vi "PCO_GetCameraDescription.vi"(8 "error in (no error)":errorcluster, 11 "Handle":u32=176713696) -> (0 "error out":errorcluster, 1 "PCO_Description_part2":T1={"wIRDESC"=1, "ZZwAlignDummy2"=0, "dwMinDelay[ns]"=0, "dwMaxDelay[ms]"=0, "dwMinDelayStep[ns]"=100, "dwMinExposure[ns]"=1000, "dwMaxExposure[ms]"=3600000, "dwMinExposureStep[ns]"=1000, "dwMinDelay[ns]"=0, "dwMaxDelay[ms]"=0, "dwMinExposureIR[ns]"=1000, "dwMaxExposureIR[ms]"=3600000, "wTimeTableDESC"=0, "wDoubleImageDESC"=1, "sMinCoolSetDESC"=0, "sMaxCoolSetDESC"=1, "sDefaultCoolSetDESC"=0, "wPowerDownModeDESC"=0, "wOffsetRegulationDESC"=1, "wColorPatternDESC"=0, "wPatternTypeDESC"=0, "wDummy1"=0, "wDummy2"=0, "wDummy3"=0, "dwGeneralCapsDESC1"=64, "dwGeneralCapsDESC2"=0}, 2 "PCO_Description_part1":T2={"wSensorTypeDESC"=16, "wSensorSubTypeDESC"=0, "wMaxHorzResStdDESC"=1392, "wMaxVertResStdDESC"=1040, "wMaxHorzResExtDESC"=800, "wMaxVertResExtDESC"=600, "wDynRes[bits]"=14, "wMaxBinHorzDESC"=4, "wBinHorzSteppingDESC"=0, "wMaxBinVertDESC"=4, "wBinVertSteppingDESC"=0, "wRoiHorStepsDESC"=0, "wRoiVertStepsDESC"=0, "wNumADCsDESC"=1} {"wSensorTypeDESC" items=["Sony ICX285AL"=16, "Sony ICX285AK"=17, "Sony ICX263AL"=32, "Sony ICX263AK"=33, "Sony ICX274AL"=48, "Sony ICX274AK"=49, "Sony ICX407AL"=64, "Sony ICX407AK"=65, "Sony ICX414AL"=80, "KAI-2000M"=272, "KAI-2001M"=288, "KAI-4010M"=304, "KAI-4011M"=306, "Micron MV13 bw"=4112, "Micron MV13 col"=4113, "Fairchild CIS2051 V1 FI"=8192, "Fairchild CIS2051 V1 BI"=8208, "Cypress RR V1 bw"=12288, "Cypress RR V1 col"=12289]}, 3 "Handle Out":u32=176713696, 4 "wConvFact[ce]":u16[](array[numeric])=[100, 150, 0, 0], 5 "return type":u32 format="%x", 6 "dwPixelRate[Hz]":u32[](array[numeric])=[12000000, 25000000, 0, 0])   [LabVIEW 2011]
uses:
  SC2_Cam64.dll
panel:
  out "PCO_Description":u16[](array[numeric])=[436, 16, 0, 1392, 1040, 800, 600, 14, 4, 0, 4, 0, 0, 0, 1, 0, 6912, 183, 30784, 381, 0, 0, 0, 0, 0, 0, 0, 0, 0, 0, 0, 0, 0, 0, 0, 0, 0, 0, 0, 0, 0, 0, 0, 0, 0, 0, 0, 0, 0, 0, 0, 0, 0, 0, 0, 0, 0, 0, 0, 0, 0, 0, 0, 0, 100, 150, 0, 0, 0, 0, 0, 0, 0, 0, 0, 0, 0, 0, 0, 0, 0, 0, 0, 0, 0, 0, 0, 0, 1, 0, 0, 0, 0, 0, 100, 0, 1000, 0, 61056, 54, 1000, 0, 0, 0, 0, 0, 1000, 0, 61056, 54, 0, 1, 0, 1, 0, 0, 1, 0, 0, 0, 0, 0, 64, 0, 0, 0, 0, 0, 0, 0, 0, 0, 0, 0, 0, 0, 0, 0, 0, 0, 0, 0, 0, 0, 0, 0, 0, 0, 0, 0, 0, 0, 0, 0, 0, 0, 0, 0, 0, 0, 0, 0, 0, 0, 0, 0, 0, 0, 0, 0, 0, 0, 0, 0, 0, 0, 0, 0, 0, 0, 0, 0, 0, 0, 0, 0, 0, 0, 0, 0, 0, 0, 0, 0, 0, 0, 0, 0, 0, 0, 0, 0, 0, 0, 0, 0, 0, 0, 0, 0, 0, 0, 0, 0, 0, 0, 0, 0, 0, 0, 0, 0, 0, 0, 0, 0, 0, 0, 0, 0, 0, 0, 0, 0, 0, 0, 0, 0, 0, 0, 0, 0, 0, 0, 0, 0, 0, 0, 0, 0, 0, 0, 0, 0, 0, 0, 0, 0, 0, 0, 0, 0, 0, 0, 0, 0, 0, 0, 0, 0, 0, 0, 0, 0, 0, 0, 0, 0, 0, 0, 0, 0, 0, 0, 0, 0, 0, 0, 0, 0, 0, 0, 0, 0, 0, 0, 0, 0, 0, 0, 0, 0, 0, 0, 0, 0, 0, 0, 0, 0, 0, 0, 0, 0, 0, 0, 0, 0, 0, 0, 0, 0, 0, 0, 0, 0, 0, 0, 0, 0, 0, 0, 0, 0, 0, 0, 0, 0, 0, 0, 0, 0, 0, 0, 0, 0, 0, 0, 0, 0, 0, 0, 0, 0, 0, 0, 0, 0, 0, 0, 0, 0, 0, 0, 0, 0, 0, 0, 0, 0, 0, 0, 0, 0, 0, 0, 0, 0, 0, 0, 0, 0, 0, 0, 0, 0, 0, 0, 0, 0, 0, 0, 0, 0, 0, 0, 0, 0, 0, 0, 0, 0, 0, 0, 0, 0, 0, 0, 0, 0, 0, 0, 0, 0, 0, 0, 0, 0, 0, 0, 0, 0, 0, 0, 0, 0, 0, 0, 0, 0, 0, 0, 0, 0, 0, 0, 0, 0, 0, 0, 0, 0, 0, 0, 0, 0, 0, 0, 0, 0, 0, 0, 0, 0, 0, 0, 0, 0, 0, 0, 0, 0, 0, 0, 0, 0, 0, 0, 0, 0, 0, 0, 0, 0, 0, 0, 0, 0, 0, 0, 0, 0, 0, 0, 0, 0, 0, 0, 0, 0, 0, 0, 0, 0, 0, 0, 0, 0, 0, 0, 0, 0, 0, 0, 0, 0, 0, 0, 0, 0, 0, 0, 0, 0, 0, 0, 0, 0, 0, 0, 0, 0, 0, 0, 0, 0, 0, 0, 0, 0, 0, 0, 0, 0, 0, 0, 0, 0, 0, 0, 0, 0, 0, 0, 0, 0, 0, 0, 0, 0, 0, 0, 0, 0, 0, 0, 0, 0, 0, 0, 0, 0, 0, 0, 0, 0, 0, 0, 0, 0, 0, 0, 0, 0, 0, 0, 0, 0, 0, 0, 0, 0, 0, 0, 0, 0, 0, 0, 0, 0, 0, 0, 0, 0, 0, 0, 0, 0, 0, 0, 0, 0, 0, 0, 0, 0, 0, 0, 0, 0, 0, 0, 0, 0, 0, 0, 0, 0, 0, 0, 0, 0, 0, 0, 0, 0, 0, 0, 0, 0, 0, 0, 0, 0, 0, 0, 0, 0, 0, 0, 0, 0, 0, 0, 0, 0, 0, 0, 0, 0, 0, 0, 0, 0, 0, 0, 0, 0, 0, 0, 0, 0, 0, 0, 0, 0, 0, 0, 0, 0, 0, 0, 0, 0, 0, 0, 0, 0, 0, 0, 0, 0, 0, 0, 0, 0, 0, 0, 0, 0, 0, 0, 0, 0, 0, 0, 0, 0, 0, 0, 0, 0, 0, 0, 0, 0, 0, 0, 0, 0, 0, 0, 0, 0, 0, 0, 0, 0, 0, 0, 0, 0, 0, 0, 0, 0, 0, 0, 0, 0]
  # "! dw Order is different!"
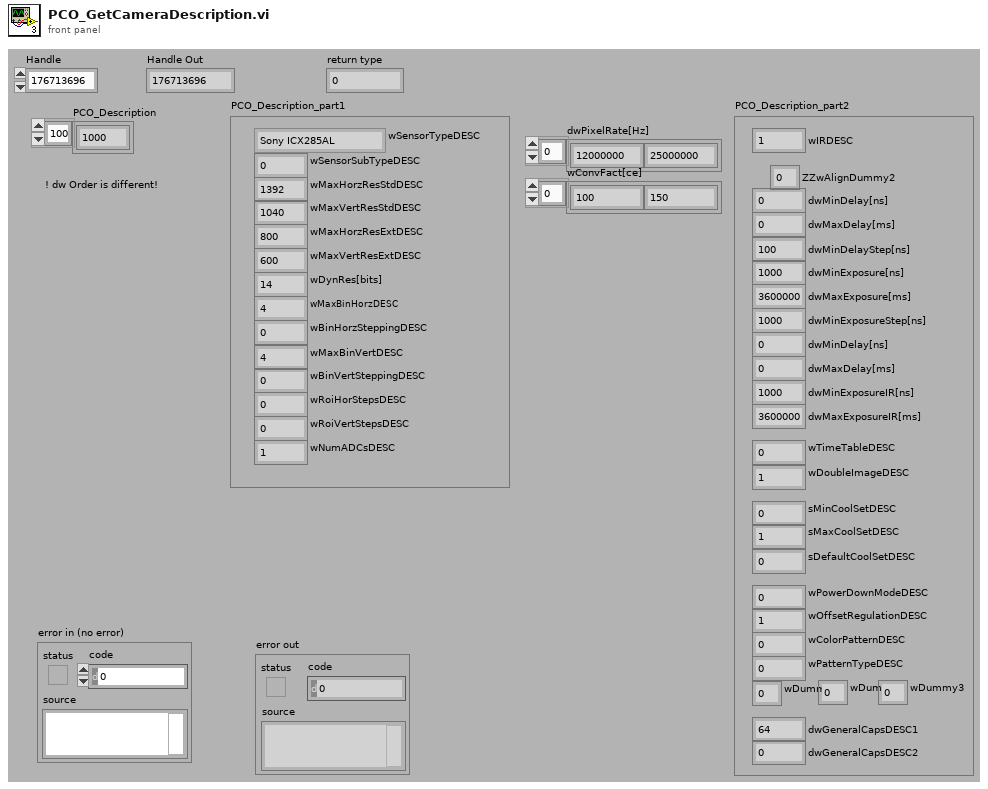
[diagram p1: front panel]
types:
  T1 = cluster{"wIRDESC":u16, "ZZwAlignDummy2":u16, "dwMinDelay[ns]":u32, "dwMaxDelay[ms]":u32, "dwMinDelayStep[ns]":u32, "dwMinExposure[ns]":u32, "dwMaxExposure[ms]":u32, "dwMinExposureStep[ns]":u32, "dwMinDelay[ns]":u32, "dwMaxDelay[ms]":u32, "dwMinExposureIR[ns]":u32, "dwMaxExposureIR[ms]":u32, "wTimeTableDESC":u16, "wDoubleImageDESC":u16, "sMinCoolSetDESC":i16, "sMaxCoolSetDESC":i16, "sDefaultCoolSetDESC":i16, "wPowerDownModeDESC":u16, "wOffsetRegulationDESC":u16, "wColorPatternDESC":u16, "wPatternTypeDESC":u16, "wDummy1":u16, "wDummy2":u16, "wDummy3":u16, "dwGeneralCapsDESC1":u32, "dwGeneralCapsDESC2":u32}
  T2 = cluster{"wSensorTypeDESC":u16, "wSensorSubTypeDESC":u16, "wMaxHorzResStdDESC":u16, "wMaxVertResStdDESC":u16, "wMaxHorzResExtDESC":u16, "wMaxVertResExtDESC":u16, "wDynRes[bits]":u16, "wMaxBinHorzDESC":u16, "wBinHorzSteppingDESC":u16, "wMaxBinVertDESC":u16, "wBinVertSteppingDESC":u16, "wRoiHorStepsDESC":u16, "wRoiVertStepsDESC":u16, "wNumADCsDESC":u16}
  T3 = cluster{"wIRDESC":u16, "ZZwAlignDummy2":u16, "dwMinDelayDESC":u32, "dwMaxDelayDESC":u32, "dwMinDelayStepDESC":u32, "dwMinExposureDESC":u32, "dwMaxExposureDESC":u32, "dwMinExposureStepDESC":u32, "dwMinDelayIRDESC":u32, "dwMaxDelayIRDESC":u32, "dwMinExposureIRDESC":u32, "dwMaxExposureIRDESC":u32, "wTimeTableDESC":u16, "wDoubleImageDESC":u16, "sMinCoolSetDESC":i16, "sMaxCoolSetDESC":i16, "sDefaultCoolSetDESC":i16, "wPowerDownModeDESC":u16, "wOffsetRegulationDESC":u16, "wColorPatternDESC":u16, "wPatternTypeDESC":u16, "wDummy1":u16, "wDummy2":u16, "wDummy3":u16, "dwGeneralCapsDESC1":u32, "dwGeneralCapsDESC2":u32}
  T4 = cluster{"wSensorTypeDESC":u16, "wSensorSubTypeDESC":u16, "wMaxHorzResStdDESC":u16, "wMaxVertResStdDESC":u16, "wMaxHorzResExtDESC":u16, "wMaxVertResExtDESC":u16, "wDynResDESC":u16, "wMaxBinHorzDESC":u16, "wBinHorzSteppingDESC":u16, "wMaxBinVertDESC":u16, "wBinVertSteppingDESC":u16, "wRoiHorStepsDESC":u16, "wRoiVertStepsDESC":u16, "wNumADCsDESC":u16}
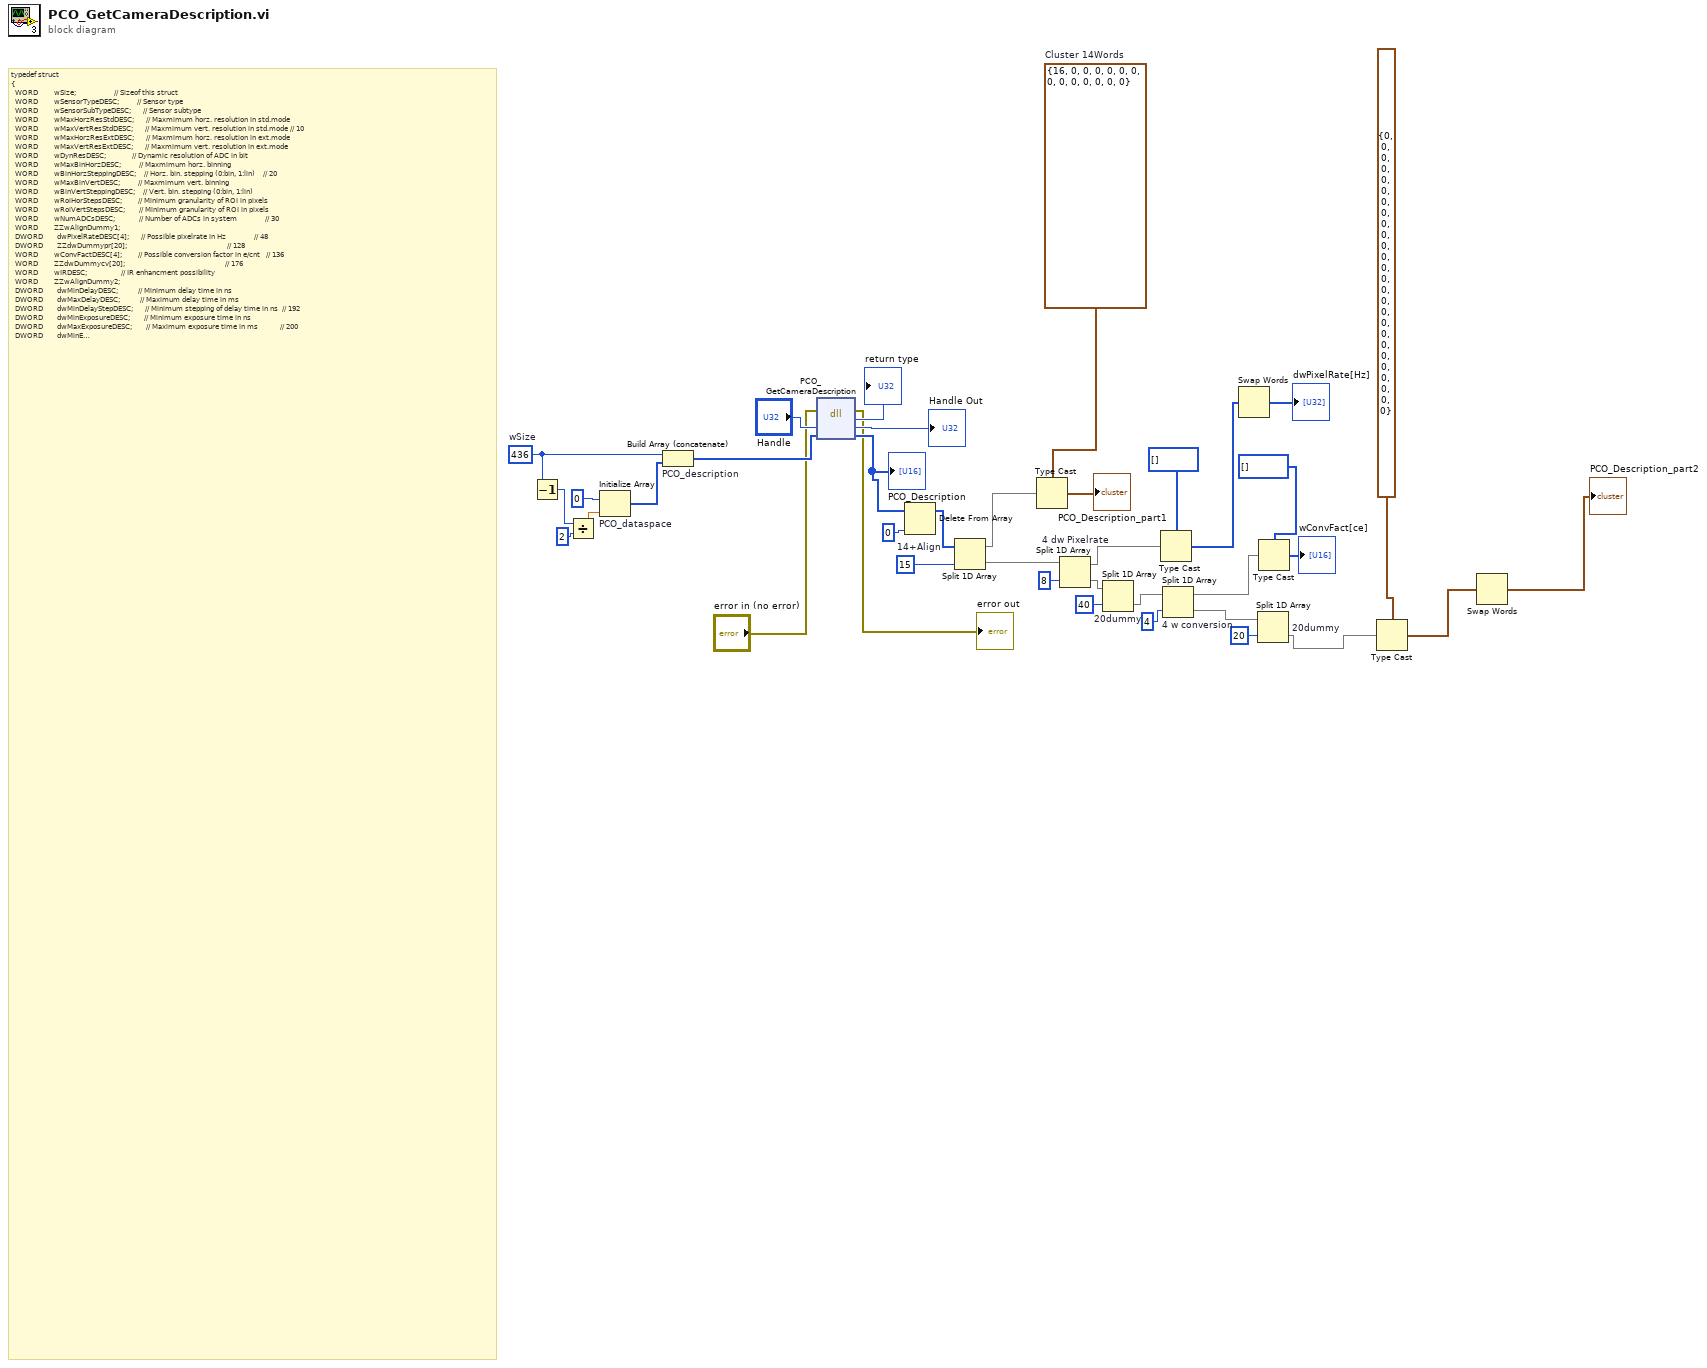
[diagram p0: block diagram]
diagram:
  w18 = T4 {"wSensorTypeDESC"=16, "wSensorSubTypeDESC"=0, "wMaxHorzResStdDESC"=0, "wMaxVertResStdDESC"=0, "wMaxHorzResExtDESC"=0, "wMaxVertResExtDESC"=0, "wDynResDESC"=0, "wMaxBinHorzDESC"=0, "wBinHorzSteppingDESC"=0, "wMaxBinVertDESC"=0, "wBinVertSteppingDESC"=0, "wRoiHorStepsDESC"=0, "wRoiVertStepsDESC"=0, "wNumADCsDESC"=0}  # Cluster 14Words
  w20 = 15  # 14+Align
  w25 = u16 436  # wSize
  # "typedef struct\n{\n  WORD        wSize;                   // Sizeof this struct\n  WORD        wSensorTypeDESC;         // Sensor type\n  WORD        wSensorSubTypeDESC;      // Sensor subtype\n  WORD        wMaxHorzResStdDESC;      // Maxmimum horz. resolution in std.mode\n  WORD        wMaxVertResStdDESC;      // Maxmimum vert. resolution in std.mode // 10\n  WORD        wMaxHorzResExtDESC;      // Maxmimum horz. resolution in ext.mode\n  WORD        wMaxVertResExtDESC;      // Maxmimum vert. resolution in ext.mode\n  WORD        wDynResDESC;             // Dynamic resolution of ADC in bit\n  WORD        wMaxBinHorzDESC;         // Maxmimum horz. binning\n  WORD        wBinHorzSteppingDESC;    // Horz. bin. stepping (0:bin, 1:lin)    // 20\n  WORD        wMaxBinVertDESC;         // Maxmimum vert. binning\n  WORD        wBinVertSteppingDESC;    // Vert. bin. stepping (0:bin, 1:lin)\n  WORD        wRoiHorStepsDESC;        // Minimum granularity of ROI in pixels\n  WORD        wRoiVertStepsDESC;       // Minimum granularity of ROI in pixels\n  WORD        wNumADCsDESC;            // Number of ADCs in system              // 30\n  WORD        ZZwAlignDummy1;\n  DWORD       dwPixelRateDESC[4];      // Possible pixelrate in Hz              // 48\n  DWORD       ZZdwDummypr[20];                                                  // 128\n  WORD        wConvFactDESC[4];        // Possible conversion factor in e/cnt   // 136\n  WORD        ZZdwDummycv[20];                                                  // 176\n  WORD        wIRDESC;                 // IR enhancment possibility\n  WORD        ZZwAlignDummy2;\n  DWORD       dwMinDelayDESC;          // Minimum delay time in ns\n  DWORD       dwMaxDelayDESC;          // Maximum delay time in ms\n  DWORD       dwMinDelayStepDESC;      // Minimum stepping of delay time in ns  // 192\n  DWORD       dwMinExposureDESC;       // Minimum exposure time in ns\n  DWORD       dwMaxExposureDESC;       // Maximum exposure time in ms           // 200\n  DWORD       dwMinExposureStepDESC;   // Minimum stepping of exposure time in ns\n  DWORD       dwMinDelayIRDESC;        // Minimum delay time in ns\n  DWORD       dwMaxDelayIRDESC;        // Maximum delay time in ms              // 212\n  DWORD       dwMinExposureIRDESC;     // Minimum exposure time in ns\n  DWORD       dwMaxExposureIRDESC;     // Maximum exposure time in ms           // 220\n  WORD        wTimeTableDESC;          // Timetable for exp/del possibility\n  WORD        wDoubleImageDESC;        // Double image mode possibility\n  SHORT       sMinCoolSetDESC;         // Minimum value for cooling\n  SHORT       sMaxCoolSetDESC;         // Maximum value for cooling\n  SHORT       sDefaultCoolSetDESC;     // Default value for cooling             // 230\n  WORD        wPowerDownModeDESC;      // Power down mode possibility\n  WORD        wOffsetRegulationDESC;   // Offset regulation possibility\n  WORD        wColorPatternDESC;       // Color pattern of color chip\n                                       // four nibbles (0,1,2,3) in word \n                                       //  ----------------- \n                                       //  | 3 | 2 | 1 | 0 |\n                                       //  ----------------- \n                                       //   \n                                       // describe row,column  2,2 2,1 1,2 1,1\n                                       // \n                                       //   column1 column2\n                                       //  ----------------- \n                                       //  |       |       |\n                                       //  |   0   |   1   |   row1\n                                       //  |       |       |\n                                       //  -----------------\n                                       //  |       |       |\n                                       //  |   2   |   3   |   row2\n                                       //  |       |       |\n                                       //  -----------------\n                                       // \n  WORD        wPatternTypeDESC;        // Pattern type of color chip\n                                       // 0: Bayer pattern RGB\n                                       // 1: Bayer pattern CMY\n  WORD        wDummy1;                 // former DSNU correction mode             // 240\n  WORD        wDummy2;                 //\n  WORD        ZZwAlignDummy3;          //\n  DWORD       dwGeneralCapsDESC1;      // General capabilities:\n                                       // Bit 0: Noisefilter available\n                                       // Bit 1: Hotpixelfilter available\n                                       // Bit 2: Hotpixel works only with noisefilter\n                                       // Bit 3: Timestamp ASCII only available (Timestamp mode 3 enabled)\n\n                                       // Bit 4: Dataformat 2x12\n                                       // Bit 5: Record Stop Event available\n                                       // Bit 6: Hot Pixel correction\n                                       // Bit 7: Ext.Exp.Ctrl. not available\n\n                                       // Bit 8: Timestamp not available\n                                       // Bit 9: Acquire mode not available\n\n                                       // Bit 31: Enhanced descriptor available\n\n  DWORD       dwGeneralCapsDESC2;      // General capabilities 2                  // 252\n  DWORD       dwReservedDESC[6];       // 32bit dummy                             // 276\n  DWORD       ZZdwDummy[40];                                                      // 436\n} PCO_Description;"
  n1 = Decrement(x=w25) -> (x-1=w24:u16)
  n2 = Divide(x=w24, y=u16 2) -> (x/y=w32:dbl)
  n3 = Initialize Array "PCO_dataspace"(u16 0 ("element"), w32) -> (w34:u16[])
  n4 = Build Array (concatenate) "PCO_description"(w25, w34) -> (w31:u16[])
  n5 = dll-call lib="C:/Program Files/colibri/Drivers/PCO.Camera/SC2_Cam*.*" fn="PCO_GetCameraDescription"(error in="error in (no error)", "Handle"="Handle", "PCO_Description"=w31) -> (error out=→"error out":errorcluster, "return type"=→"return type":u32, "Handle"=→"Handle Out":u64, "PCO_Description"=w22:u16[])  [unwired: 2 in, 1 out]
  "PCO_Description" <- w22
  n6 = Delete From Array(array=w22, index=0) -> (array with subset deleted=w21:u16[])  [unwired: 1 in, 1 out]
  n7 = Split 1D Array(array=w21, index=w20) -> (first subarray=w19:u16[], second subarray=w16:u16[])
  n8 = Type Cast(type=w18, x=w19) -> (*(type *) &x=→"PCO_Description_part1":T4)
  n9 = Split 1D Array "4 dw Pixelrate"(array=w16, index=8) -> (first subarray=w15:u16[], second subarray=w5:u16[])
  n10 = Split 1D Array "20dummy"(array=w5, index=40) -> (second subarray=w4:u16[])  [unwired: 1 out]
  n11 = Type Cast(type=u32[] [], x=w15) -> (*(type *) &x=w9:u32[])
  n12 = Split 1D Array "4 w conversion"(array=w4, index=4) -> (first subarray=w28:u16[], second subarray=w27:u16[])
  n13 = Swap Words(1:w9) -> (0:→"dwPixelRate[Hz]":u32[])
  n14 = Split 1D Array "20dummy"(array=w27, index=20) -> (second subarray=w11:u16[])  [unwired: 1 out]
  n15 = Type Cast(type=u16[] [], x=w28) -> (*(type *) &x=→"wConvFact[ce]":u16[])
  n16 = Type Cast(type=T3 {"wIRDESC"=0, "ZZwAlignDummy2"=0, "dwMinDelayDESC"=0, "dwMaxDelayDESC"=0, "dwMinDelayStepDESC"=0, "dwMinExposureDESC"=0, "dwMaxExposureDESC"=0, "dwMinExposureStepDESC"=0, "dwMinDelayIRDESC"=0, "dwMaxDelayIRDESC"=0, "dwMinExposureIRDESC"=0, "dwMaxExposureIRDESC"=0, "wTimeTableDESC"=0, "wDoubleImageDESC"=0, "sMinCoolSetDESC"=0, "sMaxCoolSetDESC"=0, "sDefaultCoolSetDESC"=0, "wPowerDownModeDESC"=0, "wOffsetRegulationDESC"=0, "wColorPatternDESC"=0, "wPatternTypeDESC"=0, "wDummy1"=0, "wDummy2"=0, "wDummy3"=0, "dwGeneralCapsDESC1"=0, "dwGeneralCapsDESC2"=0} ("Cluster 2"), x=w11) -> (*(type *) &x=w7:T3)
  n17 = Swap Words(1:w7) -> (0:→"PCO_Description_part2":T3)
